vi "DROPBEAR_Model_Updating_Online.vi"(8 "error in (no error)":errorcluster, 11 "DROPBEAR_Model_Updating in":refnum<class "DROPBEAR_Model_Updating.lvclass">) -> (0 "error out":errorcluster, 3 "DROPBEAR_Model_Updating out":refnum<class "DROPBEAR_Model_Updating.lvclass">, 4 "looping":bool)   [LabVIEW 2021, in "DROPBEAR_Model_Updating.lvclass"]
uses:
  DROPBEAR_Model_Updating.lvclass
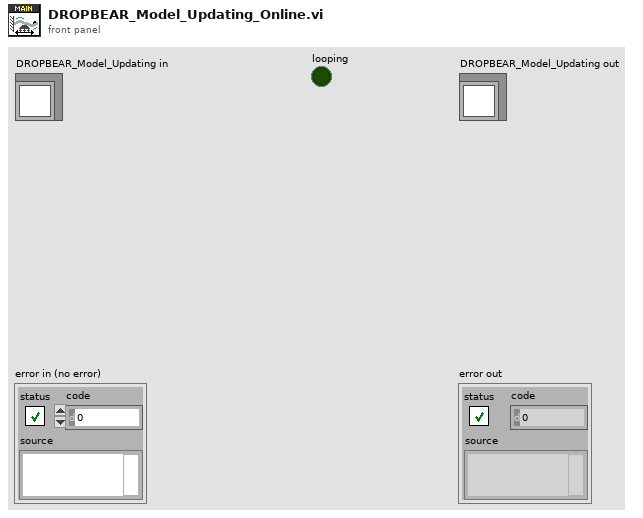
[diagram p1: front panel]
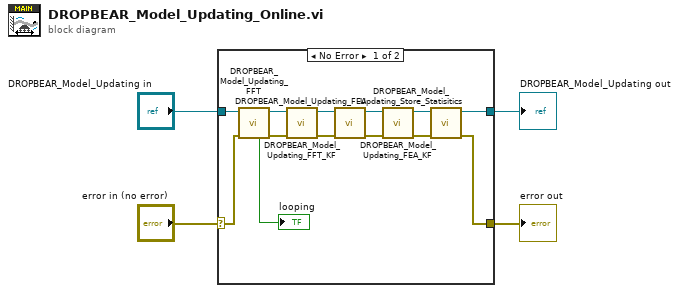
[diagram p0: block diagram]
diagram:
  n1 = case shown="No Error" "error in (no error)" {
    selector: "error in (no error)" -> [w7 w19]
    tunnel: [w6 w19] -> w3
    tunnel: [w8 w18] -> w1
    tunnel: "DROPBEAR_Model_Updating in" -> [w17 w18]
    frame No Error {
      n2 = call-dynamic "DROPBEAR_Model_Updating_FFT.vi"("error in (no error)"=w7, "DROPBEAR_Model_Updating in"=w17) -> ("error out"=w15:errorcluster, "DROPBEAR_Model_Updating out"=w16:refnum<class "DROPBEAR_Model_Updating.lvclass">, "looping"=→"looping":bool)  [unwired: 7 in]
      n3 = call-dynamic "DROPBEAR_Model_Updating_FFT_KF.vi"("error in (no error)"=w15, "DROPBEAR_Model_Updating in"=w16) -> ("error out"=w13:errorcluster, "DROPBEAR_Model_Updating out"=w14:refnum<class "DROPBEAR_Model_Updating.lvclass">)  [unwired: 8 in]
      n4 = call-dynamic "DROPBEAR_Model_Updating_FEA.vi"("error in (no error)"=w13, "DROPBEAR_Model_Updating in"=w14) -> ("error out"=w11:errorcluster, "DROPBEAR_Model_Updating out"=w12:refnum<class "DROPBEAR_Model_Updating.lvclass">)  [unwired: 8 in]
      n5 = call-dynamic "DROPBEAR_Model_Updating_FEA_KF.vi"("error in (no error)"=w11, "DROPBEAR_Model_Updating in"=w12) -> ("error out"=w9:errorcluster, "DROPBEAR_Model_Updating out"=w10:refnum<class "DROPBEAR_Model_Updating.lvclass">)  [unwired: 8 in]
      n6 = call-dynamic "DROPBEAR_Model_Updating_Store_Statisitics.vi"("error in (no error)"=w9, "DROPBEAR_Model_Updating in"=w10) -> ("error out"=w6:errorcluster, "DROPBEAR_Model_Updating out"=w8:refnum<class "DROPBEAR_Model_Updating.lvclass">)  [unwired: 8 in]
    }
    frame Error {
    }
  }
  "error out" <- w3
  "DROPBEAR_Model_Updating out" <- w1
